vi "Open.vi"(8 "error in":errorcluster, 9 "parameters":variant, 10 "file path":path, 11 "repository in":refnum<class "CustomDeviceRepo.lvclass">) -> (0 "error out":errorcluster, 2 "invalid?":bool, 3 "repository out":refnum<class "CustomDeviceRepo.lvclass">)   [LabVIEW 2015, in "CustomDeviceRepo.lvclass"]
doc: "Loads the saved information of the repo. It could load multiple files at the same time. An option to add file versioning could be included in the files, and the code to manage changes would be in this VI."
uses:
  CustomDeviceRepo.lvclass
  CustomDeviceRepo.lvclass/CustomDeviceRepo.ctl
  VeriStand Custom Device XML Parser.lvlib
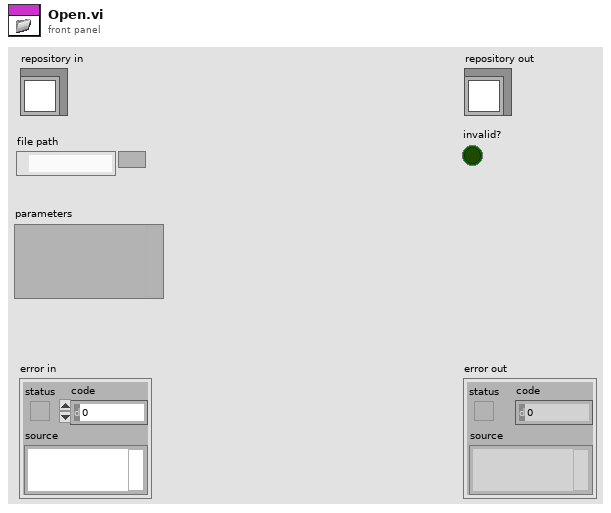
[diagram p1: front panel]
types:
  T1 = typedef "VeriStand Custom Device XML Parser.lvlib/Main Custom Device Properties.ctl" = cluster{"CD Name":string, "Version":string, "Max Occurrences":i32, "Device Type":enum16{"Asynchronous", "Inline HW Interface", "Inline Model Interface", "Inline Timing and Sync", "Asynchronous Timing and Sync"}, "Main Page GUID":string}
  T2 = typedef "VeriStand Custom Device XML Parser.lvlib/Initialization VI Properties.ctl" = cluster{"Execution":T3, "Path":T4, "Type":enum16{"Action", "VI"}, "Position":enum16{"centered", "mouse pointer"}}
  T3 = typedef "VeriStand Custom Device XML Parser.lvlib/Execution Types.ctl" = enum16{"silent", "modal", "floating", "default"}
  T4 = typedef "VeriStand Custom Device XML Parser.lvlib/Path Cluster.ctl" = cluster{"Path":path, "Path Type":enum16{"Absolute", "To Base", "To Common Doc Dir", "To Application Data Dir"}}
  T5 = typedef "VeriStand Custom Device XML Parser.lvlib/Timing Source Properties.ctl" = cluster{"Has Timing Source Capability":bool, "Source Distribution":T6}
  T6 = typedef "VeriStand Custom Device XML Parser.lvlib/Timing Source Source Distribution Properties.ctl" = cluster{"Supported Target":T7, "Source":T4, "Real Time System Destination":string, "Version":string}[]
  T7 = typedef "VeriStand Custom Device XML Parser.lvlib/Supported Targets.ctl" = enum16{"All", "Pharlap", "VxWorks", "Windows", "Linux_32_ARM", "Linux_x64", "PharlapWindows", "PharlapVxWorks", "VxWorksWindows"}
  T8 = typedef "VeriStand Custom Device XML Parser.lvlib/Custom Device Source Distribution Properties.ctl" = cluster{"Source":T4, "Real Time System Destination":string, "Supported Target":T7}[]
  T9 = typedef "VeriStand Custom Device XML Parser.lvlib/Help File Properties.ctl" = cluster{"Item to Launch":T4, "Section":string, "File Type":enum16{"chm", "other"}}
  T10 = typedef "VeriStand Custom Device XML Parser.lvlib/Button Properties.ctl" = cluster{"ID":string, "Glyph":T4, "Button Type":T11, "Referenced GUID":string, "Button Text":string, "Caption":string, "Tip Strip":string, "Documentation":string, "Dependency":T12}
  T11 = typedef "VeriStand Custom Device XML Parser.lvlib/Button Type.ctl" = enum16{"Action", "Dialog", "Page", "Notification", "Separator"}
  T12 = typedef "VeriStand Custom Device XML Parser.lvlib/Dependency Properties.ctl" = cluster{"File Path Control":path, "Path Type":enum16{"Absolute", "To Base", "To Common Doc Dir", "To Application Data Dir"}, "Behavior":enum16{"Static", "Dynamic"}}
  T13 = typedef "VeriStand Custom Device XML Parser.lvlib/RuntTimeMenu Properties.ctl" = cluster{"GUID":string, "Execution":T3, "MinNrOfChilds":u32, "Name":string, "Item to Launch":T4, "Dependency":T12, "Custom Population":T4, "Menu Item Type":enum16{"Action", "VI", "Separator", "Custom"}, "Behavior":enum16{"Nothing", "Open Front Panel"}, "Position":enum16{"Centered", "Mouse Pointer"}}
  T14 = cluster{"Cluster":cluster{"Name":string, "Disallow Renaming":bool, "Delete Protection":bool, "Exlcude from Alphabetical order":bool, "Allow Multi-Selection":bool, "GUID":string, "Parent GUIDs":string[], "Glyph":T4, "Inactive Glyph":T4, "Broken Glyph":T4, "Item to Launch":T4, "Additional Information":string, "Copy":enum16{"copy", "disabled"}, "Paste":enum16{"Create", "CreatIfNotExists_GUID", "CreatIfNotExists_Name", "Replace", "Dialog"}, "Help":T9}, "Cluster":cluster{"Action VI On Delete":T4, "Action VI On Load":T4, "Action VI On Paste":T4, "Action VI On Target Type Change":T4, "Action VI On Delete Request":T4, "Action VI On Compile":T4, "Action VI On System Shutdown":T4, "Action VI On Save":T4, "Action VI On Download":T4}, "Button List":T10[], "Run Time Menu":T13[]}[]
  T15 = typedef "VeriStand Custom Device XML Parser.lvlib/Dependencies Properties.ctl" = cluster{"ForceDownload":bool, "RealTimeSystemDestination":string, "Path Properties":T4, "Supported Target":T7, "Version":string, "SupportedTargetSpecified":bool}
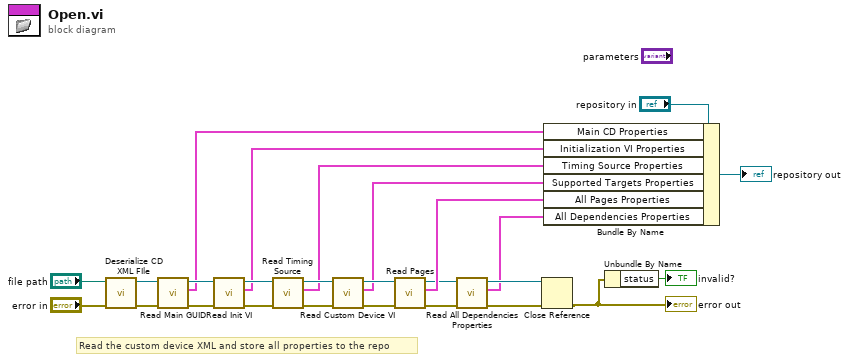
[diagram p0: block diagram]
diagram:
  # "Read the custom device XML and store all properties to the repo"
  n1 = call "Deserialize CD XML FIle.vi"("Error In"="error in", "XML Path"="file path") -> ("Error Out"=w24:errorcluster, "Custom Device .NET Ref Out"=w23:refnum<k24>)  [unwired: 8 in]
  n2 = call "Read Main GUID.vi"("Error In"=w24, "Custom Device .NET Ref In"=w23) -> ("Error out"=w17:errorcluster, "Main CD Properties"=w10:T1, "Custom Device .NET Ref Out"=w18:refnum<k24>)  [unwired: 7 in]
  n3 = call "Read Init VI.vi"("Error In"=w17, "Custom Device .NET Ref In"=w18) -> ("Error Out"=w16:errorcluster, "Initialization VI Properties"=w9:T2, "Custom Device .NET Ref Out"=w15:refnum<k24>)  [unwired: 7 in]
  n4 = call "Read Timing Source.vi"("Error In"=w16, "Custom Device .NET Ref In"=w15) -> ("Error Out"=w14:errorcluster, "Timing Source Properties"=w8:T5, "Custom Device .NET Ref Out"=w13:refnum<k24>)  [unwired: 7 in]
  n5 = call "Read Custom Device VI.vi"("Error In"=w14, "Custom Device .NET Ref In"=w13) -> ("Error Out"=w11:errorcluster, "Supported Targets Properties"=w7:T8, "Custom Device .NET Ref In"=w12:refnum<k24>)  [unwired: 7 in]
  n6 = call "Read Pages.vi"("Error In"=w11, "Custom Device Page .NET Ref In"=w12) -> ("Error Out"=w5:errorcluster, "All Pages Properties"=w6:T14, "Custom Device Page .NET Ref Out"=w3:refnum<k24>)  [unwired: 7 in]
  n7 = call "Read All Dependencies Properties.vi"("Error In"=w5, "Custom Device .NET Ref In"=w3) -> ("Error Out"=w4:errorcluster, "All Dependencies Properties"=w1:T15[], "Custom Device .NET Ref Out"=w2:refnum<k24>)  [unwired: 7 in]
  n8 = Close Reference(reference=w2, error in (no error)=w4) -> (error out=w20:errorcluster)
  "error out" <- w20
  n9 = Bundle By Name(cluster="repository in", "Main CD Properties"=w10, "Initialization VI Properties"=w9, "Timing Source Properties"=w8, "Supported Targets Properties"=w7, "All Pages Properties"=w6, "All Dependencies Properties"=w1) -> (→"repository out":refnum<class "CustomDeviceRepo.lvclass">)
  n10 = Unbundle By Name(w20) -> ("status"=→"invalid?":bool)
